vi "Destructor.vi"(8 "ErrorIn":errorcluster, 11 "OpenCVFaceDetectionIn":refnum<class "OpenCVFaceDetection.lvclass">) -> (0 "ErrorOut":errorcluster, 3 "OpenCVFaceDetectionOut":refnum<class "OpenCVFaceDetection.lvclass">)   [LabVIEW 2021, in "OpenCVFaceDetection.lvclass"]
doc: "Called at the destruction of the object. Use this to clear references or perform action to tidy up the object."
uses:
  OpenCVFaceDetection.lvclass
  OpenCVFaceDetection.lvclass/OpenCVFaceDetection.ctl
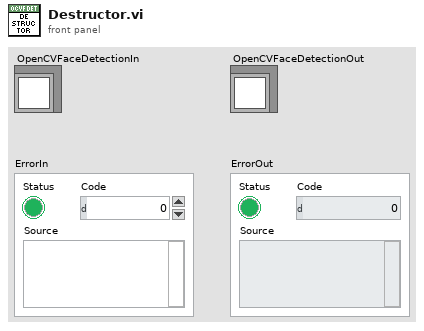
[diagram p1: front panel]
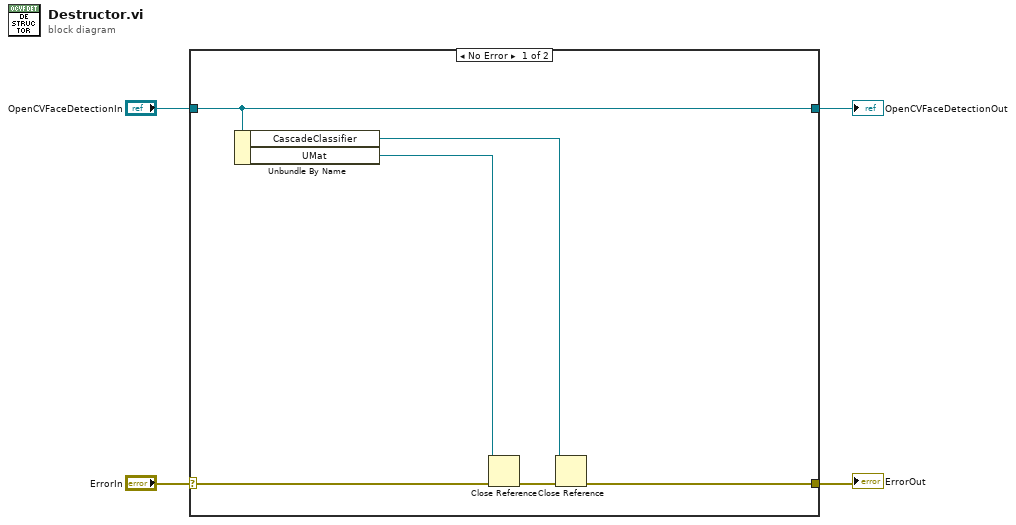
[diagram p0: block diagram]
diagram:
  n1 = case shown="No Error" "ErrorIn" {
    selector: "ErrorIn" -> [w10 w12]
    tunnel: [w8 w12] -> w3
    tunnel: [w7 w11] -> w1
    tunnel: "OpenCVFaceDetectionIn" -> [w7 w11]
    frame No Error {
      n2 = Unbundle By Name(w7) -> ("CascadeClassifier"=w5:refnum<k24>, "UMat"=w6:refnum<k24>)
      n3 = Close Reference(reference=w6, error in (no error)=w10) -> (error out=w9:errorcluster)
      n4 = Close Reference(reference=w5, error in (no error)=w9) -> (error out=w8:errorcluster)
    }
    frame Error {
    }
  }
  "ErrorOut" <- w3
  "OpenCVFaceDetectionOut" <- w1
